vi "next chunk -- init.vi"(5 "temperature":dbl=-1.0, 8 "chunks":T9={"start F (Hz)"=1400000.0, "stop F (Hz)"=3000000.0, "total number of points"=6000, "chunk size"=10, "freq step (Hz)"=400.0, "update rate (Hz)"=250.0, "adaptive parameters"={"peaks are known -- parameters"={"Def Gamma (kHz)"=0.5, "dV"=17.0, "time in Gamma (sec)"=7.0, "phi-star"=0.0, "all peaks (kHz)"=[], "delta t (sec)"=22.0, "default step (Hz)"=0.0, "all gamma (kHz)"=[564.0, 649.0, 987.0, 1133.0, 1214.0, 1585.0, 1763.0, 1823.0, 1880.0, 1899.0, 2032.0, 2138.0, 2221.0, 2270.0, 2350.0, 2456.0, 2580.0, 2634.0, 2831.0, 2960.0, 2965.0, 3131.0, 3328.0, 3469.0, 3553.0, 0.0, 3615.0, 3734.0, 0.0, 0.0, 0.0, 4236.0, 4300.0, 4331.0], "peaks OK"=FALSE, "gamma OK"=FALSE, "near omega (kHz)"=0.0, "near gamma (kHz)"=0.0, "min step (Hz)"=10000.0, "max step(Hz)"=0.01, "min gamma (kHz)"=0.01, "all time in gamma (sec)"=[], "time in gamma OK"=FALSE, "time-in-gamma mode"=enum."same for all"}, "find peak - parameters"={"wavepacket"={"R"=0.5, "wave number"=17.0, "delta k"=7.0, "radii vector"=[], "radial section"=[], "wave vector"=22.0, "wavepacket is"=TRUE}, "number of grid points"=70, "decimation threshold"=1, "Voltage range"=0.1, "target freq step"=20.0, "target spot size"=0.05, "factor"=1.0, "another factor"=1.0, "analyze last # sec"=3, "scale factor"=3}}, "total sweep time (sec)"=24.0, "chunk time (sec)"=0.04, "spot size (V)"=5.8152639158694506e-05, "uniform freq step (Hz)"=266.6666666666667, "next start freq (Hz)"=1412960.0000000002} {"next start freq (Hz)" format="%#9_8f"; "uniform freq step (Hz)" format="%#_3f"; "spot size (V)" format="%#_2f"; "adaptive parameters"."find peak - parameters"."wavepacket"."delta k" format="%#_3f"; "adaptive parameters"."find peak - parameters"."wavepacket"."wave number" format="%#_3f"; "adaptive parameters"."find peak - parameters"."wavepacket"."R" format="%#_3f"; "freq step (Hz)" format="%#4_4f"; "stop F (Hz)" format="%#_3f"; "start F (Hz)" format="%#_3f"}, 9 "sweep settings":T1={"time gap (min) "=0.0, "Bypass error dialog"=TRUE, "range factor"=1.05, "min gamma(kHz)"=0.005, "max step(Hz)"=1.05, "min step(Hz)"=0.005, "save freq units"=enum."Hz", "Zero signal?"=FALSE, "time in Gamma --OK"=FALSE, "scan mode"=enum."predictive", "power control mode "=enum."power vs Temp", "time-in-gamma mode"=enum."same for all"}, 10 "adaptive parameters":T5={"peaks are known -- parameters"={"Def Gamma (kHz)"=0.5, "dV"=17.0, "time in Gamma (sec)"=7.0, "phi-star"=0.0, "all peaks (kHz)"=[], "delta t (sec)"=22.0, "default step (Hz)"=0.0, "all gamma (kHz)"=[564.0, 649.0, 987.0, 1133.0, 1214.0, 1585.0, 1763.0, 1823.0, 1880.0, 1899.0, 2032.0, 2138.0, 2221.0, 2270.0, 2350.0, 2456.0, 2580.0, 2634.0, 2831.0, 2960.0, 2965.0, 3131.0, 3328.0, 3469.0, 3553.0, 0.0, 3615.0, 3734.0, 0.0, 0.0, 0.0, 4236.0, 4300.0, 4331.0], "peaks OK"=FALSE, "gamma OK"=FALSE, "near omega (kHz)"=0.0, "near gamma (kHz)"=0.0, "min step (Hz)"=10000.0, "max step(Hz)"=0.01, "min gamma (kHz)"=0.01, "all time in gamma (sec)"=[], "time in gamma OK"=FALSE, "time-in-gamma mode"=enum."same for all"}, "find peak - parameters"={"wavepacket"={"R"=0.5, "wave number"=17.0, "delta k"=7.0, "radii vector"=[], "radial section"=[], "wave vector"=22.0, "wavepacket is"=TRUE}, "number of grid points"=70, "decimation threshold"=1, "Voltage range"=0.1, "target freq step"=20.0, "target spot size"=0.05, "factor"=1.0, "another factor"=1.0, "analyze last # sec"=3, "scale factor"=3}} {"find peak - parameters"."wavepacket"."delta k" format="%#_3f"; "find peak - parameters"."wavepacket"."wave number" format="%#_3f"; "find peak - parameters"."wavepacket"."R" format="%#_3f"}, 11 "RUS settings":T10={"NI-DAQ lockin settings"={"Samples per sine wave"=0, "Sine waves per freq step"=0, "Output Representation"=enum."Real/Imaginary", "Low-pass filter"=enum."Butterworth", "Ranges and couplings "=[]}, "Fast swep settings"={"Update rate (Hz)"=250.0, "Start F, Hz"=200000.0, "Stop F"=1700000.0, "Number of points"=30000, "Amplitude"=2.1, "Init&amplitude"=TRUE, "IF"=1000.0, "Time constant"=0.1}, "Pre-sweep delay, s"=0.0, "Lockin mode"=enum."NI-DAQ", "SR Lockin"="GPIB0::10::INSTR", "DAQmx Device"="Dev3", "Clock Multiplier"=64, "Fast Sweep Data Out"={"DO clock task"="", "DO task"="", "Update clock task"="", "DAQ lockin task"="", "Pre-sweep counter task"=""}, "Lockin Range, V"=0.0, "F Array"=[], "Freq. update clock terminal"="", "DO Clock Rate (Hz)"=5000000.0, "ADC clock terminal"="/PFI4", "Pre-sweep counter terminal"="", "Samples per read"=10, "DO clock terminal"="", "Pre-sweep points"=0, "F points per write"=1000, "Total sweep time, s"=0.0, "Initial SYNTH phase"=0.0, "Record IF"=FALSE, "Save data settings"={"Save data"=TRUE, "Data Root Path"=path "", "File Prefix"="", "File Format"=enum."ASCII", "Save column names"=TRUE, "File Comments"="<Description of the current file>", "User/Prj"="<User Name/Project Description>"}, "Data file path"=path "", "New data user event"=refnum, "Stop user event"=refnum, "Number of channels"=1, "Auto-phase"=FALSE, "RP Transeiver"=refnum} {"Lockin Range, V" format="%#_6e"; "Fast swep settings"."IF" format="%#_6p"; "Fast swep settings"."Amplitude" min=0.0 max=2.5; "Fast swep settings"."Number of points" format="%.0p"; "Fast swep settings"."Stop F" format="%#_6p"; "Fast swep settings"."Start F, Hz" format="%#_6p"; "Fast swep settings"."Update rate (Hz)" format="%0.2f"; "NI-DAQ lockin settings"."Ranges and couplings"."Coupling" items=["default"=-1, "RSE"=10083, "NRSE"=10078, "Differential"=10106, "Pseudodifferential"=12529]}) -> (0 "chunks out":T9={"start F (Hz)"=1400000.0, "stop F (Hz)"=3000000.0, "total number of points"=6000, "chunk size"=10, "freq step (Hz)"=400.0, "update rate (Hz)"=250.0, "adaptive parameters"={"peaks are known -- parameters"={"Def Gamma (kHz)"=0.5, "dV"=17.0, "time in Gamma (sec)"=7.0, "phi-star"=0.0, "all peaks (kHz)"=[], "delta t (sec)"=22.0, "default step (Hz)"=0.0, "all gamma (kHz)"=[564.0, 649.0, 987.0, 1133.0, 1214.0, 1585.0, 1763.0, 1823.0, 1880.0, 1899.0, 2032.0, 2138.0, 2221.0, 2270.0, 2350.0, 2456.0, 2580.0, 2634.0, 2831.0, 2960.0, 2965.0, 3131.0, 3328.0, 3469.0, 3553.0, 0.0, 3615.0, 3734.0, 0.0, 0.0, 0.0, 4236.0, 4300.0, 4331.0], "peaks OK"=FALSE, "gamma OK"=FALSE, "near omega (kHz)"=0.0, "near gamma (kHz)"=0.0, "min step (Hz)"=10000.0, "max step(Hz)"=0.01, "min gamma (kHz)"=0.01, "all time in gamma (sec)"=[], "time in gamma OK"=FALSE, "time-in-gamma mode"=enum."same for all"}, "find peak - parameters"={"wavepacket"={"R"=0.5, "wave number"=17.0, "delta k"=7.0, "radii vector"=[], "radial section"=[], "wave vector"=22.0, "wavepacket is"=TRUE}, "number of grid points"=70, "decimation threshold"=1, "Voltage range"=0.1, "target freq step"=20.0, "target spot size"=0.05, "factor"=1.0, "another factor"=1.0, "analyze last # sec"=3, "scale factor"=3}}, "total sweep time (sec)"=24.0, "chunk time (sec)"=0.04, "spot size (V)"=5.8152639158694506e-05, "uniform freq step (Hz)"=266.6666666666667, "next start freq (Hz)"=1412960.0000000002} {"next start freq (Hz)" format="%#9_8f"; "uniform freq step (Hz)" format="%#_3f"; "spot size (V)" format="%#_2f"; "adaptive parameters"."find peak - parameters"."wavepacket"."delta k" format="%#_3f"; "adaptive parameters"."find peak - parameters"."wavepacket"."wave number" format="%#_3f"; "adaptive parameters"."find peak - parameters"."wavepacket"."R" format="%#_3f"; "freq step (Hz)" format="%#4_4f"; "stop F (Hz)" format="%#_3f"; "start F (Hz)" format="%#_3f"}, 2 "adaptive parameters out":T5={"peaks are known -- parameters"={"Def Gamma (kHz)"=0.5, "dV"=17.0, "time in Gamma (sec)"=7.0, "phi-star"=0.0, "all peaks (kHz)"=[], "delta t (sec)"=22.0, "default step (Hz)"=0.0, "all gamma (kHz)"=[564.0, 649.0, 987.0, 1133.0, 1214.0, 1585.0, 1763.0, 1823.0, 1880.0, 1899.0, 2032.0, 2138.0, 2221.0, 2270.0, 2350.0, 2456.0, 2580.0, 2634.0, 2831.0, 2960.0, 2965.0, 3131.0, 3328.0, 3469.0, 3553.0, 0.0, 3615.0, 3734.0, 0.0, 0.0, 0.0, 4236.0, 4300.0, 4331.0], "peaks OK"=FALSE, "gamma OK"=FALSE, "near omega (kHz)"=0.0, "near gamma (kHz)"=0.0, "min step (Hz)"=10000.0, "max step(Hz)"=0.01, "min gamma (kHz)"=0.01, "all time in gamma (sec)"=[], "time in gamma OK"=FALSE, "time-in-gamma mode"=enum."same for all"}, "find peak - parameters"={"wavepacket"={"R"=0.5, "wave number"=17.0, "delta k"=7.0, "radii vector"=[], "radial section"=[], "wave vector"=22.0, "wavepacket is"=TRUE}, "number of grid points"=70, "decimation threshold"=1, "Voltage range"=0.1, "target freq step"=20.0, "target spot size"=0.05, "factor"=1.0, "another factor"=1.0, "analyze last # sec"=3, "scale factor"=3}} {"find peak - parameters"."wavepacket"."delta k" format="%#_3f"; "find peak - parameters"."wavepacket"."wave number" format="%#_3f"; "find peak - parameters"."wavepacket"."R" format="%#_3f"}, 4 "next chunk action":T4=enum."next chunk - peaks are known", 6 "next chunk init action":T4=enum."next chunk - peaks are known")   [LabVIEW 2016]
uses:
  single sweep - frequency chunks.ctl
  single sweep - adaptive parameters.ctl
  next chunk -- parameters.ctl
  time in gamma mode control.ctl
  find peak -- parameters.ctl
  wavepacket.ctl
  resonant_ultrasound/Libraries/RUS/Controls/RUS settings.ctl
  NHMFL_Core/Libraries/Red Pitaya/RP Core/RP Transceiver/RP Transceiver.lvclass
  resonant_ultrasound/Libraries/RUS/Controls/RUS NI-DAQ Lockin Settings.ctl
  resonant_ultrasound/Libraries/RUS/Controls/Sweep settings.ctl
  resonant_ultrasound/Libraries/RUS/Controls/Lockin mode.ctl
  NHMFL_Core/Libraries/File/Controls/Save data settings.ctl
  NHMFL_Core/Libraries/File/Controls/File formats.ctl
  next chunk -- action.ctl
  adaptive sweep UI controls.ctl
  next chunk -- algorithm.ctl
  Q - not nan -- real.vi
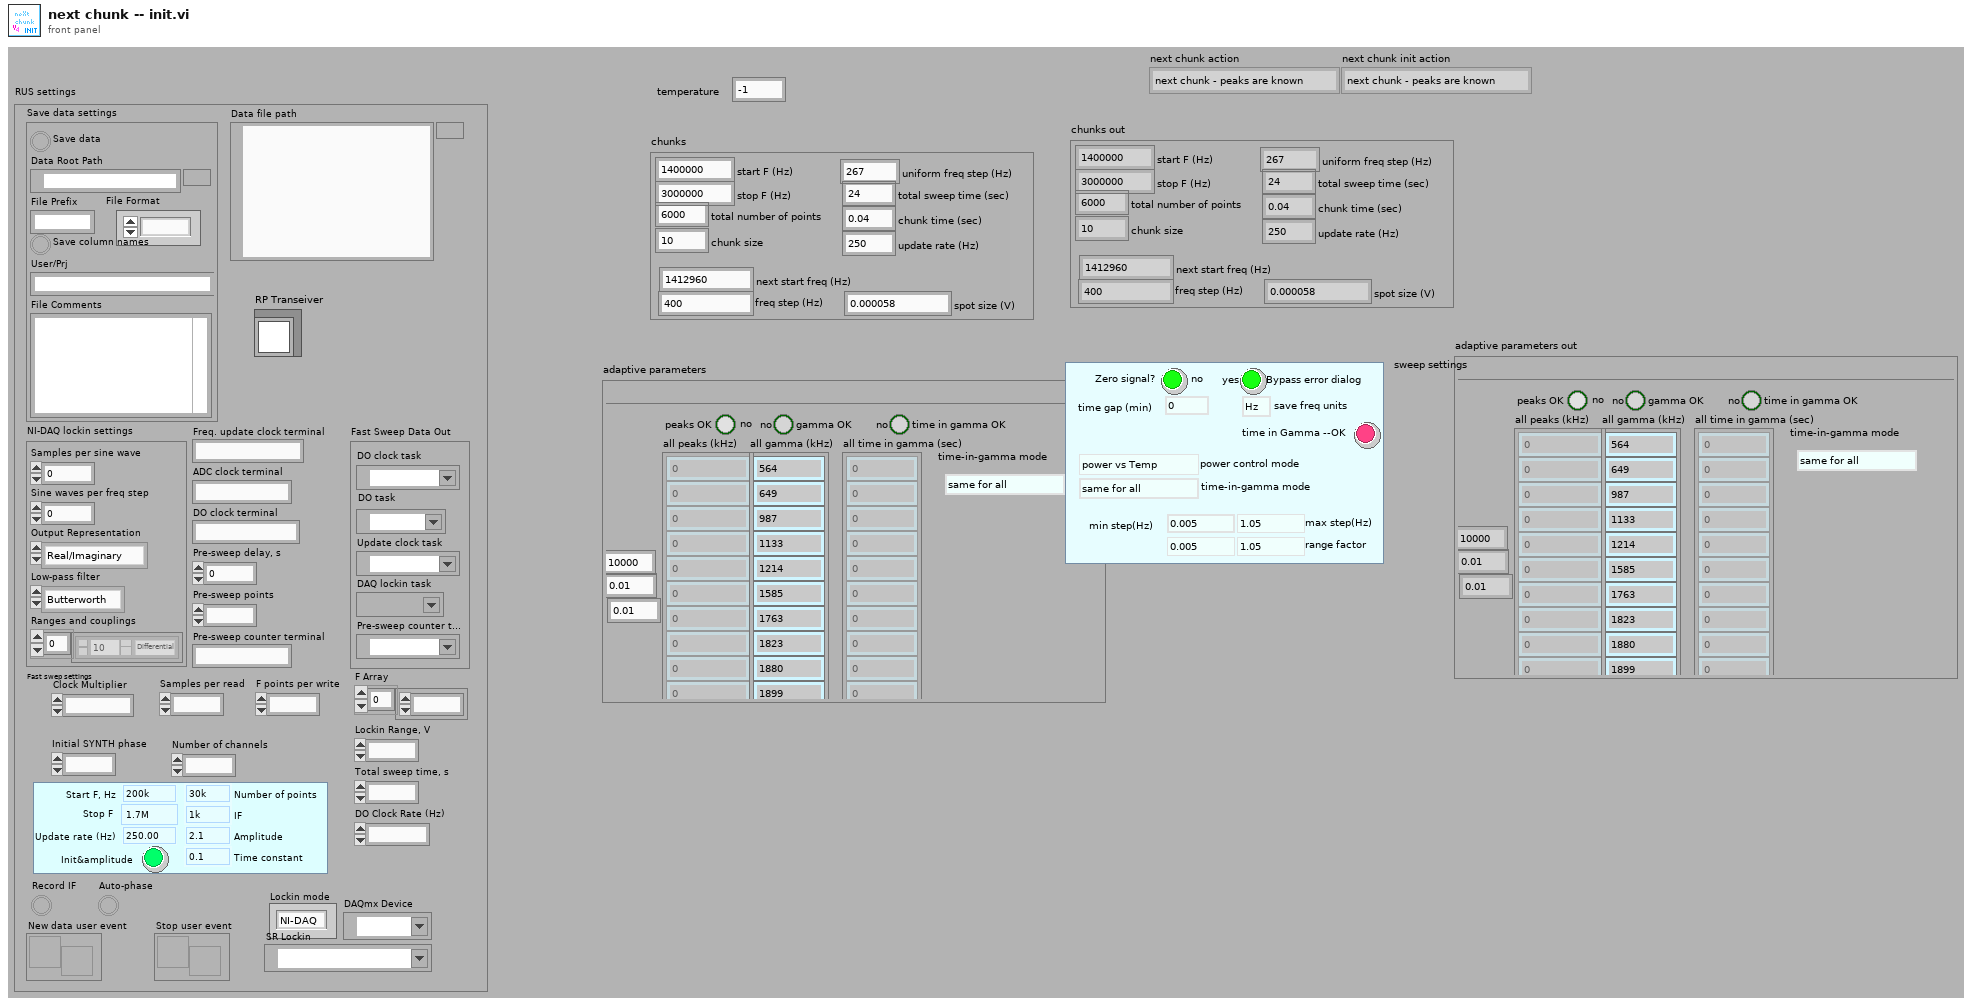
[diagram p1: front panel]
types:
  T1 = typedef "adaptive sweep UI controls.ctl" = cluster{"time gap (min) ":dbl, "Bypass error dialog":bool, "range factor":dbl, "min gamma(kHz)":dbl, "max step(Hz)":dbl, "min step(Hz)":dbl, "save freq units":enum16{"kHz", "Hz"}, "Zero signal?":bool, "time in Gamma --OK":bool, "scan mode":T2, "power control mode ":enum16{"power vs Temp", "power vs Time", "none"}, "time-in-gamma mode":T3}
  T2 = typedef "next chunk -- algorithm.ctl" = enum16{"peak position is known", "uniform", "predictive"}
  T3 = typedef "time in gamma mode control.ctl" = enum16{"same for all", "each one different", "uniform scan"}
  T4 = typedef "next chunk -- action.ctl" = enum16{"empty", "init - uniform", "next chunk - uniform", "next chunk - peaks are known", "init - peaks are known", ""}
  T5 = typedef "single sweep - adaptive parameters.ctl" = cluster{"peaks are known -- parameters":T6, "find peak - parameters":T7}
  T6 = typedef "next chunk -- parameters.ctl" = cluster{"Def Gamma (kHz)":dbl, "dV":dbl, "time in Gamma (sec)":dbl, "phi-star":dbl, "all peaks (kHz)":dbl[], "delta t (sec)":dbl, "default step (Hz)":dbl, "all gamma (kHz)":dbl[], "peaks OK":bool, "gamma OK":bool, "near omega (kHz)":dbl, "near gamma (kHz)":dbl, "min step (Hz)":dbl, "max step(Hz)":dbl, "min gamma (kHz)":dbl, "all time in gamma (sec)":dbl[], "time in gamma OK":bool, "time-in-gamma mode":T3}
  T7 = typedef "find peak -- parameters.ctl" = cluster{"wavepacket":T8, "number of grid points":i32, "decimation threshold":i32, "Voltage range":dbl, "target freq step":dbl, "target spot size":dbl, "factor":dbl, "another factor":dbl, "analyze last # sec":i32, "scale factor":i32}
  T8 = typedef "wavepacket.ctl" = cluster{"R":dbl, "wave number":dbl, "delta k":dbl, "radii vector":dbl[], "radial section":cdb[], "wave vector":dbl, "wavepacket is":bool}
  T9 = typedef "single sweep - frequency chunks.ctl" = cluster{"start F (Hz)":dbl, "stop F (Hz)":dbl, "total number of points":i32, "chunk size":i32, "freq step (Hz)":dbl, "update rate (Hz)":dbl, "adaptive parameters":T5, "total sweep time (sec)":dbl, "chunk time (sec)":dbl, "spot size (V)":dbl, "uniform freq step (Hz)":dbl, "next start freq (Hz)":dbl}
  T10 = typedef "RUS settings.ctl" = cluster{"NI-DAQ lockin settings":T11, "Fast swep settings":T12, "Pre-sweep delay, s":dbl, "Lockin mode":T13, "SR Lockin":refnum<visa-resource-name>, "DAQmx Device":tag, "Clock Multiplier":i32, "Fast Sweep Data Out":cluster{"DO clock task":refnum<k21>, "DO task":refnum<k21>, "Update clock task":refnum<k21>, "DAQ lockin task":refnum<k21>, "Pre-sweep counter task":refnum<k21>}, "Lockin Range, V":sgl, "F Array":dbl[], "Freq. update clock terminal":string, "DO Clock Rate (Hz)":dbl, "ADC clock terminal":string, "Pre-sweep counter terminal":string, "Samples per read":i32, "DO clock terminal":string, "Pre-sweep points":i32, "F points per write":i32, "Total sweep time, s":dbl, "Initial SYNTH phase":dbl, "Record IF":bool, "Save data settings":T14, "Data file path":path, "New data user event":refnum<user-event>, "Stop user event":refnum<user-event>, "Number of channels":i32, "Auto-phase":bool, "RP Transeiver":refnum<class "RP Transceiver.lvclass">}
  T11 = typedef "RUS NI-DAQ Lockin Settings.ctl" = cluster{"Samples per sine wave":i32, "Sine waves per freq step":i32, "Output Representation":enum16{"Real/Imaginary", "Polar"}, "Low-pass filter":enum16{"No filtering", "Butterworth", "Bessel"}, "Ranges and couplings ":cluster{"Range":dbl, "Coupling":i32}[]}
  T12 = typedef "Sweep settings.ctl" = cluster{"Update rate (Hz)":dbl, "Start F, Hz":dbl, "Stop F":dbl, "Number of points":i32, "Amplitude":dbl, "Init&amplitude":bool, "IF":dbl, "Time constant":dbl}
  T13 = typedef "Lockin mode.ctl" = enum16{"SRS", "NI-DAQ", "Pitaya"}
  T14 = typedef "Save data settings.ctl" = cluster{"Save data":bool, "Data Root Path":path, "File Prefix":string, "File Format":T15, "Save column names":bool, "File Comments":string, "User/Prj":string}
  T15 = typedef "File formats.ctl" = enum16{"TDMS", "ASCII", "BINARY"}
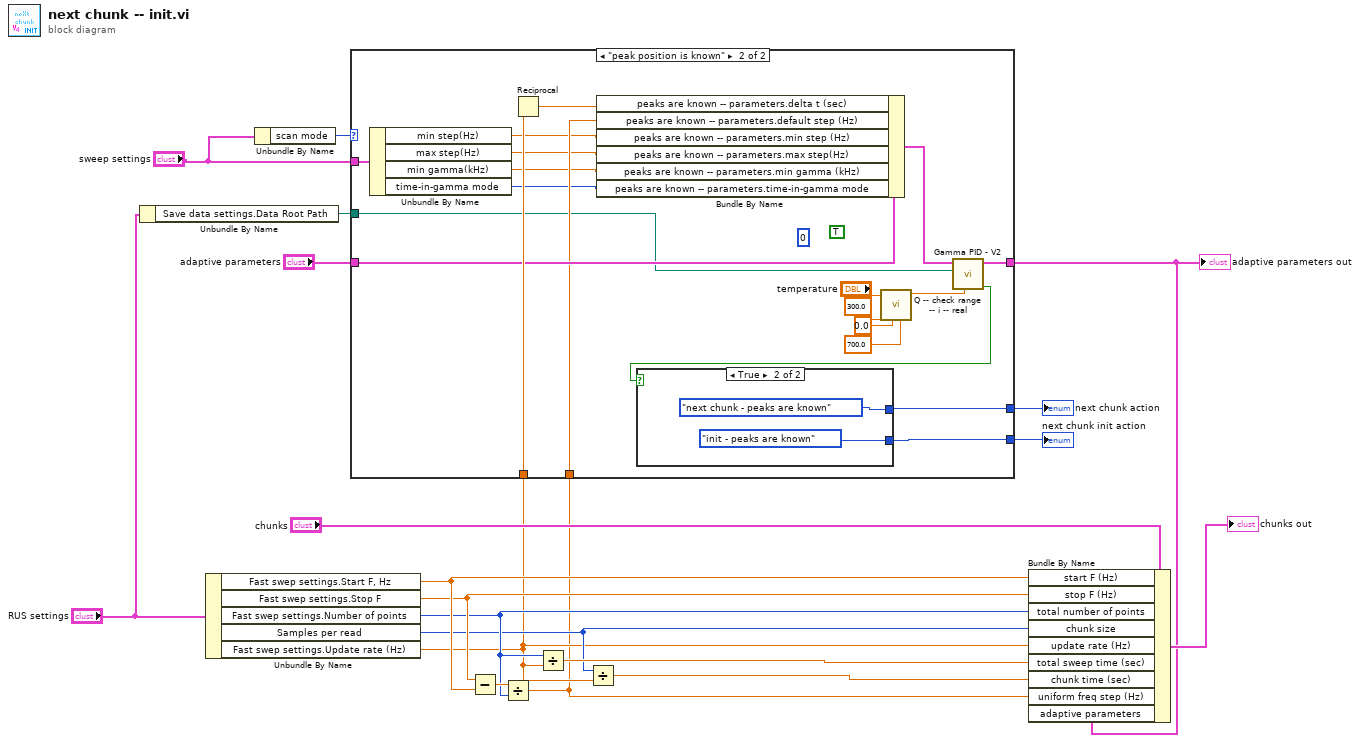
[diagram p0: block diagram]
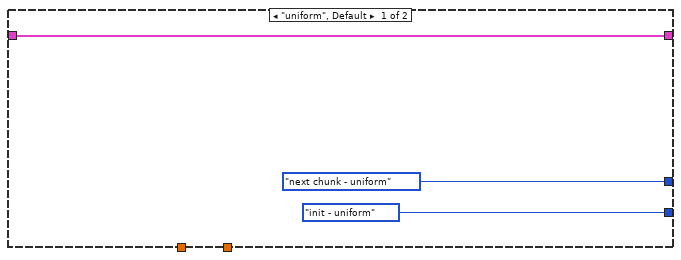
[diagram p2: hidden frame]
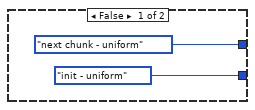
[diagram p3: hidden frame]
diagram:
  n1 = Unbundle By Name("RUS settings") -> ("Save data settings.Data Root Path"=w6:path)
  n2 = Unbundle By Name("RUS settings") -> ("Fast swep settings.Start F, Hz"=w18:dbl, "Fast swep settings.Stop F"=w17:dbl, "Fast swep settings.Number of points"=w15:i32, "Samples per read"=w14:i32, "Fast swep settings.Update rate (Hz)"=w10:dbl)
  n3 = Unbundle By Name("sweep settings") -> ("scan mode"=w3:T2)
  n4 = Subtract(x=w17, y=w18) -> (x-y=w16:dbl)
  n5 = Divide(x=w16, y=w15) -> (x/y=w8:dbl)
  n6 = case shown="\"peak position is known\"" w3 {
    tunnel: [next_chunk_--_action."init - uniform" ("next chunk action") w25] -> w1
    tunnel: [next_chunk_--_action."next chunk - uniform" ("next chunk action") w26] -> w2
    tunnel: w10 -> [_ w41]
    tunnel: "adaptive parameters" -> [w20 w40]
    tunnel: [w20 w27] -> w5
    tunnel: w8 -> [_ w35]
    tunnel: w6 -> [_ w33]
    tunnel: "sweep settings" -> [_ w31]
    frame "uniform", Default {
    }
    frame "peak position is known" {
      (unwired) 0 ("index")
      (unwired) TRUE ("control gamma PID?")
      n7 = Unbundle By Name(w31) -> ("min step(Hz)"=w30:dbl, "max step(Hz)"=w29:dbl, "min gamma(kHz)"=w28:dbl, "time-in-gamma mode"=w23:T3)
      n8 = Reciprocal(x=w41) -> (1/x=w42:dbl)
      n9 = Bundle By Name(cluster=w40, "peaks are known -- parameters.delta t (sec)"=w42, "peaks are known -- parameters.default step (Hz)"=w35, "peaks are known -- parameters.min step (Hz)"=w30, "peaks are known -- parameters.max step(Hz)"=w29, "peaks are known -- parameters.min gamma (kHz)"=w28, "peaks are known -- parameters.time-in-gamma mode"=w23) -> (w34:T5)
      n10 = call "Q -- check range -- i -- real.vi"("upper"=700.0, "lower"=0.0, "default"=300.0, "number"="temperature") -> ("number in range"=w32:dbl)  [unwired: 5 in, 2 out]
      n11 = call "Gamma PID - V2.vi"("nonzero temperature"=w32, "sweep folder path"=w33, "adaptive parameters"=w34) -> ("Peaks OK"=w24:bool, "adaptive parameters out"=w27:T5)  [unwired: 7 in]
      n12 = case shown="True" w24 {
        tunnel: [next_chunk_--_action."next chunk - uniform" ("next chunk action") next_chunk_--_action."next chunk - peaks are known" ("next chunk action")] -> w26
        tunnel: [next_chunk_--_action."init - uniform" ("next chunk action") next_chunk_--_action."init - peaks are known" ("next chunk action")] -> w25
        frame False {
        }
        frame True {
        }
      }
    }
  }
  "adaptive parameters out" <- w5
  "next chunk action" <- w2
  "next chunk init action" <- w1
  n13 = Divide(x=w15, y=w10) -> (x/y=w19:dbl)
  n14 = Divide(x=w14, y=w10) -> (x/y=w11:dbl)
  n15 = Bundle By Name(cluster="chunks", "start F (Hz)"=w18, "stop F (Hz)"=w17, "total number of points"=w15, "chunk size"=w14, "update rate (Hz)"=w10, "total sweep time (sec)"=w19, "chunk time (sec)"=w11, "uniform freq step (Hz)"=w8, "adaptive parameters"=w5) -> (→"chunks out":T9)
